vi "WeightingCheckNew.vi"() -> ()   [LabVIEW 2012]
uses:
  <vilib>/addons/database/Auxilliary.llb/DB Tools Cursor Type.ctl
  <vilib>/addons/database/Connection.llb/DB Tools Open Connec (Path).vi
  <vilib>/Utility/file.llb/Read From Spreadsheet File (string).vi
  <vilib>/addons/database/Connection.llb/Conn Execute.vi
  <vilib>/addons/database/Recordset.llb/Rec Fetch Integer Data (R).vi
  <vilib>/addons/database/Recordset.llb/Rec Destroy - Connection.vi
  <vilib>/Utility/file.llb/Write To Spreadsheet File (string).vi
  <vilib>/addons/database/NI_Database_API.lvlib
panel:
  out "WrongDate":bool
  in  "Cluster":T1
  out "after substring":string
  out "Wrong RC":bool
  out "STD Weight Check":bool
  out "Total Check":bool
  out "data":i32
  out "Pass Check":bool
  out "ProdLine":bool
  out "error out":errorcluster
  out "filenames":string[](array[string])
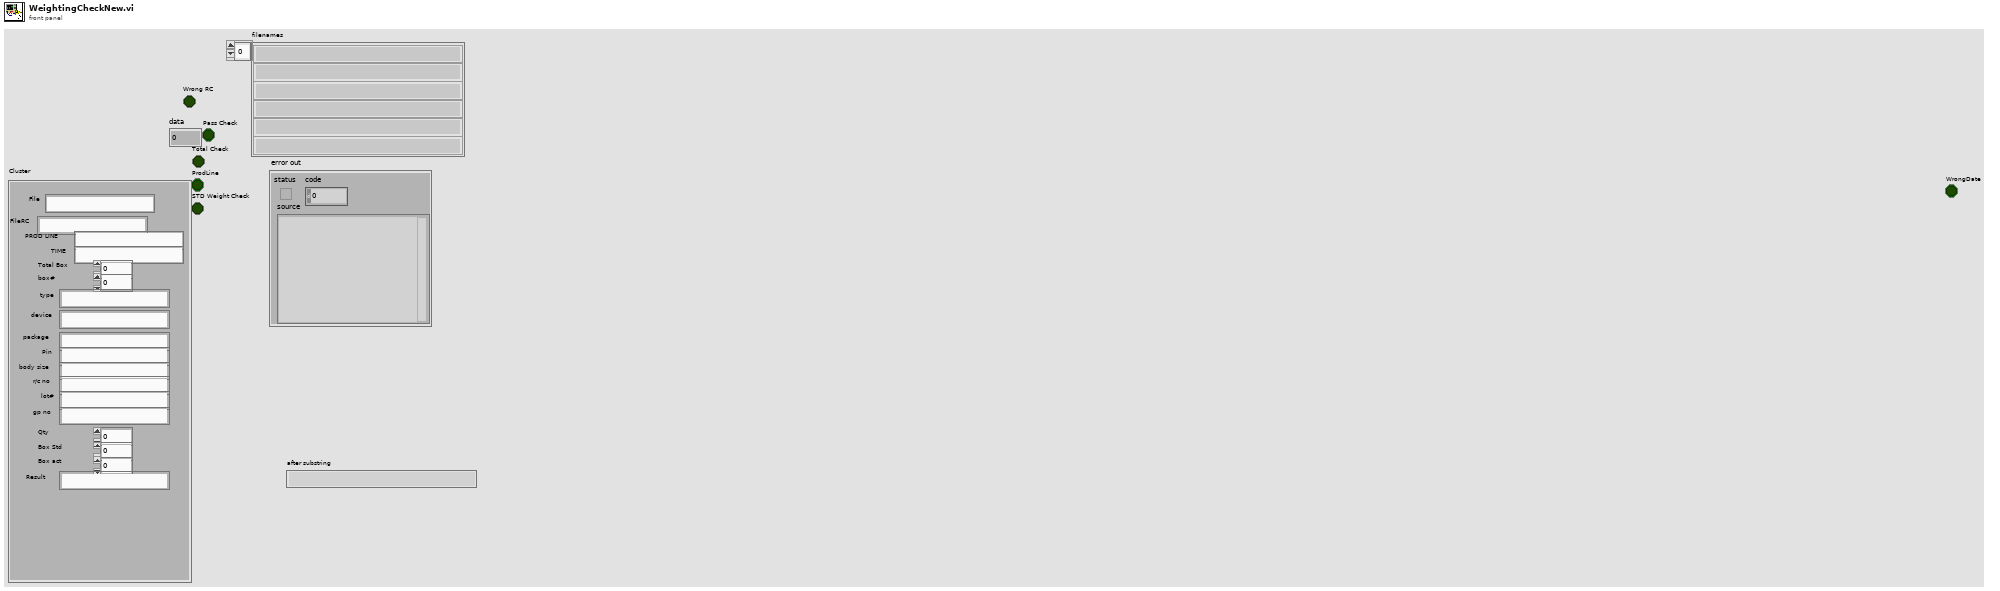
[diagram p1: front panel]
types:
  T1 = cluster{"File":string, "FileRC":string, "PROD LINE ":string, "TIME":string, "Total Box":dbl, "box#":dbl, "type":string, "device":string, "package":string, "Pin ":string, "body size":string, "r/c no":string, "lot#":string, "gp no":string, "Qty":dbl, "Box Std":dbl, "Box act":dbl, "Result":string}
  T2 = typedef "NI_Database_API.lvlib/DB Tools Cursor Type.ctl" = enum16{"forward-only", "keyset", "dynamic", "static"}
  T3 = typedef "NI_Database_API.lvlib/Conn ObjectReference.ctl" = refnum<k1>
  T4 = typedef "NI_Database_API.lvlib/Rec ObjectReference.ctl" = refnum<k1>
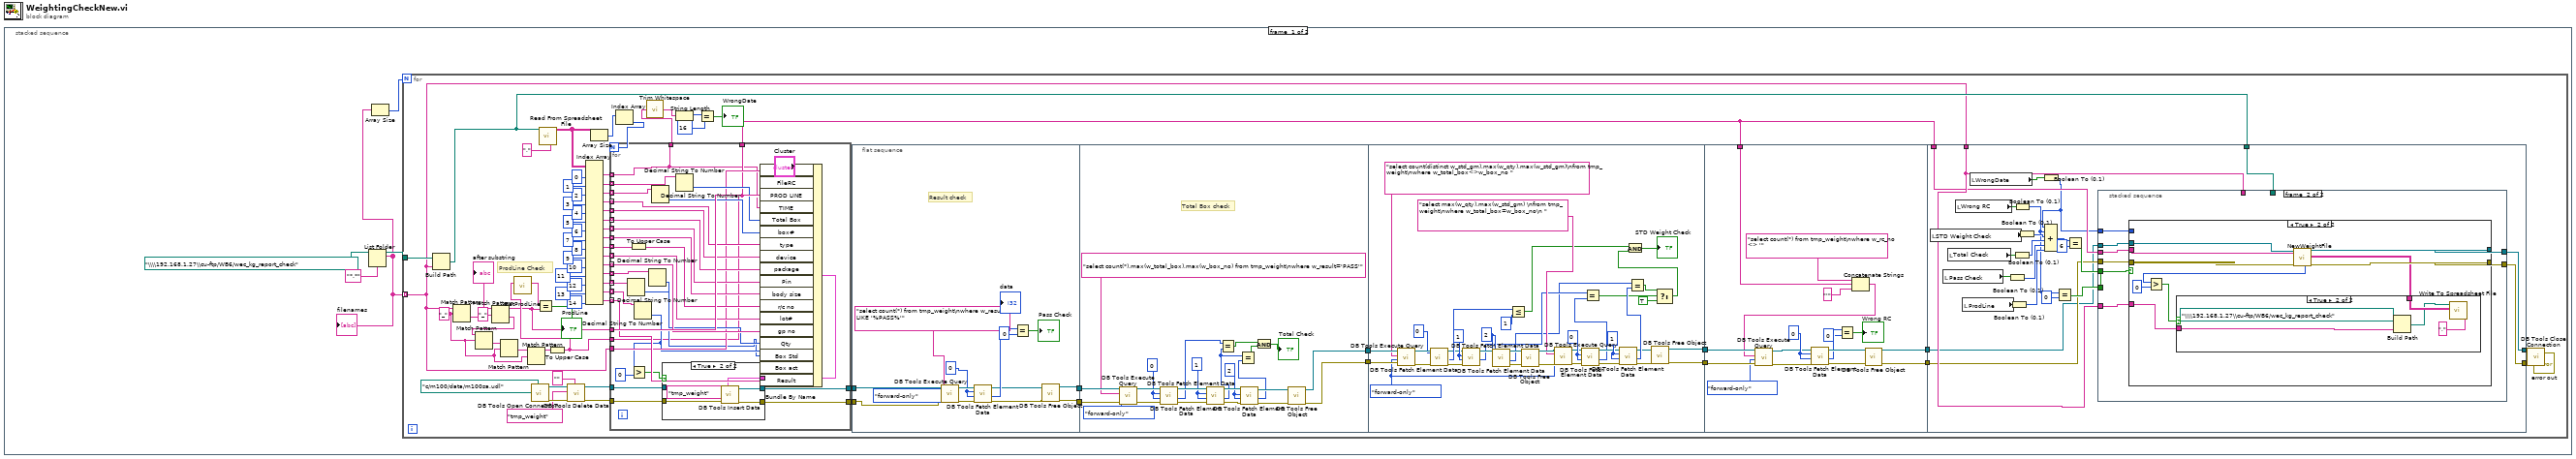
[diagram p0: block diagram]
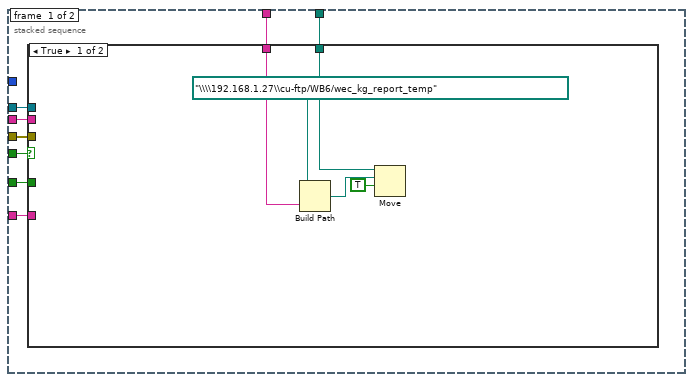
[diagram p2: hidden frame]
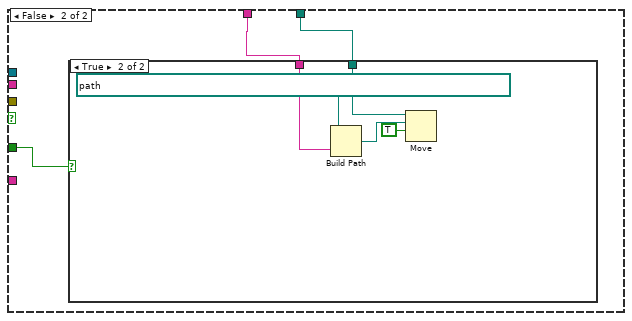
[diagram p3: hidden frame]
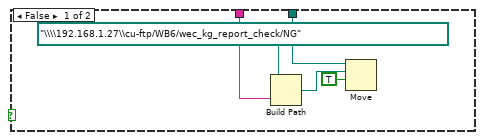
[diagram p4: hidden frame]
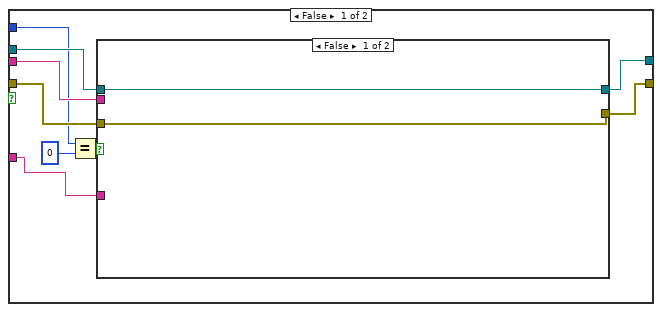
[diagram p5: hidden frame]
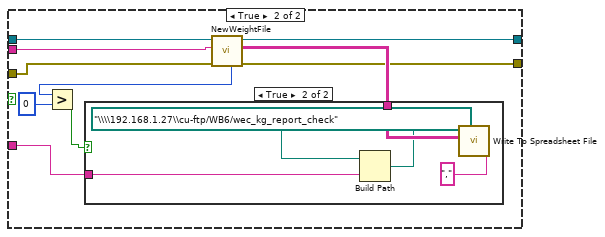
[diagram p6: hidden frame]
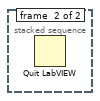
[diagram p10: hidden frame]
diagram:
  n1 = stacked-sequence {
    frame #0 {
      n2 = List Folder(path=path "\\\\192.168.1.27\\cu-ftp/WB6/wec_kg_report_check", pattern="*.*") -> (path out=w3:path, filenames=w1:string[])  [unwired: 2 in, 2 out]
      "filenames" <- w1
      n3 = Array Size(array=w1) -> (size(s)=w2:i32)
      n4 = for {
        N: w2 -> [_]
        tunnel: w3 -> [w61]
        tunnel: w1 -> [w15] mode=indexing
        w56 = "_" ("regular expression")
        # "ProdLine Check"
        n5 = Build Path(base path=w61, name or relative path=w15) -> (appended path=w16:path)
        n6 = Match Pattern(string=w15, regular expression=w56) -> (after substring=w59:string)  [unwired: 1 in, 3 out]
        "after substring" <- w59
        n7 = Match Pattern(string=w59, regular expression="_") -> (before substring=w24:string, after substring=w55:string)  [unwired: 1 in, 2 out]
        n8 = Match Pattern(string=w55, regular expression=w56) -> (after substring=w58:string)  [unwired: 1 in, 3 out]
        n9 = Match Pattern(string=w58, regular expression=w56) -> (after substring=w57:string)  [unwired: 1 in, 3 out]
        n10 = Match Pattern(string=w57, regular expression=w56) -> (before substring=w54:string)  [unwired: 1 in, 3 out]
        n11 = call-poly <vilib>:"DB Tools Open Connection.vi"("connection information"=path "c:/m100/data/m100sa.udl") -> ("error out"=w35:errorcluster, "connection reference"=w36:T3)  [unwired: 7 in]
        n12 = call-poly <vilib>:"Read From Spreadsheet File.vi"("delimiter (\\t)"="," ("delimiter (\\t)"), "file path (dialog if empty)"=w16) -> ("all rows"=w77:string[][])  [unwired: 5 in, 4 out]
        n13 = To Upper Case(1:w54) -> (0:w26:string)
        n14 = call "GetProdLine.vi"("Lotno"=w26) -> ("ProdLine"=w25:string)  [unwired: 10 in]
        n15 = Equal?(x=w25, y=w24) -> (x = y?=→"ProdLine":bool)
        n16 = call <vilib>:"DB Tools Delete Data.vi"("condition"="", "error in (no error)"=w35, "table"="tmp_weight", "connection reference"=w36) -> ("error out"=w33:errorcluster, "connection reference out"=w34:T3)  [unwired: 6 in]
        n17 = Index Array(array=w77, index (col) #1=0 ("disabled index (col)"), index (col) #2=1 ("index (col)"), index (col) #3=2 ("index (col)"), index (col) #4=3 ("index (col)"), index (col) #5=4 ("index (col)"), index (col) #6=5 ("index (col)"), index (col) #7=6 ("index (col)"), index (col) #8=7 ("index (col)"), index (col) #9=8 ("index (col)"), index (col) #10=9 ("index (col)"), index (col) #11=10 ("index (col)"), index (col) #12=11 ("index (col)"), index (col) #13=12 ("index (col)"), index (col) #14=13 ("index (col)"), index (col) #15=14 ("index (col)")) -> (element #1=w69:string[], element #2=w67:string[], element #3=w66:string[], element #4=w65:string[], element #5=w64:string[], element #6=w63:string[], element #7=w62:string[], element #8=w47:string[], element #9=w44:string[], element #10=w43:string[], element #11=w42:string[], element #12=w41:string[], element #13=w40:string[], element #14=w39:string[], element #15=w38:string[])  [unwired: 15 in]
        n18 = Array Size(array=w77) -> (size(s)=w78:i32[])
        n19 = Index Array(array=w78) -> (element=w68:i32)  [unwired: 1 in]
        n20 = for {
          N: w68 -> [_]
          tunnel: w69 -> [w272] mode=indexing
          tunnel: w67 -> [w302] mode=indexing
          tunnel: w66 -> [w298] mode=indexing
          tunnel: w65 -> [w296] mode=indexing
          tunnel: w64 -> [w295] mode=indexing
          tunnel: w63 -> [w294] mode=indexing
          tunnel: w62 -> [w293] mode=indexing
          tunnel: w47 -> [w292] mode=indexing
          tunnel: w44 -> [w303] mode=indexing
          tunnel: w43 -> [w290] mode=indexing
          tunnel: w42 -> [w289] mode=indexing
          tunnel: w41 -> [w288] mode=indexing
          tunnel: w40 -> [w286] mode=indexing
          tunnel: w39 -> [w285] mode=indexing
          tunnel: w38 -> [w284] mode=indexing
          tunnel: w26 -> [w273]
          tunnel: w15 -> [w283]
          tunnel: w24 -> [w300]
          tunnel: w34 -> [w282]
          tunnel: w33 -> [w281]
          tunnel: [w280] -> w30
          tunnel: [w279] -> w29
          tunnel: [w273] -> w12
          tunnel: [w272] -> w6
          n21 = Decimal String To Number(string=w286) -> (number=w274:i32)  [unwired: 2 in, 1 out]
          n22 = To Upper Case(1:w303) -> (0:w291:string)
          n23 = Decimal String To Number(string=w285) -> (number=w277:i32)  [unwired: 2 in, 1 out]
          n24 = Greater?(x=w277, y=0) -> (0:w275:bool)
          n25 = Decimal String To Number(string=w288) -> (number=w287:i32)  [unwired: 2 in, 1 out]
          n26 = Decimal String To Number(string=w298) -> (number=w297:i32)  [unwired: 2 in, 1 out]
          n27 = Decimal String To Number(string=w302) -> (number=w299:i32)  [unwired: 2 in, 1 out]
          n28 = Bundle By Name(cluster="Cluster", "File"=w283, "FileRC"=w273, "PROD LINE"=w300, "TIME"=w272, "Total Box"=w299, "box#"=w297, "type"=w296, "device"=w295, "package"=w294, "Pin"=w293, "body size"=w292, "r/c no"=w291, "lot#"=w290, "gp no"=w289, "Qty"=w287, "Box Std"=w274, "Box act"=w277, "Result"=w284) -> (w278:T1)
          n29 = case shown="True" w275 {
            tunnel: w282 -> [w305 w311]
            tunnel: w281 -> [w304 w310]
            tunnel: [w305 w309] -> w280
            tunnel: [w304 w308] -> w279
            tunnel: w278 -> [_ w307]
            frame False {
            }
            frame True {
              n30 = call <vilib>:"DB Tools Insert Data.vi"("data"=w307, "error in (no error)"=w310, "table"="tmp_weight", "connection reference"=w311) -> ("error out"=w308:errorcluster, "connection reference out"=w309:T3)  [unwired: 6 in]
            }
          }
        }
        n31 = call <vilib>:"Trim Whitespace.vi"("string"=w6) -> ("trimmed string"=w7:string)  [unwired: 1 in]
        n32 = String Length(string=w7) -> (length=w10:i32)
        n33 = Equal?(x=w10, y=16) -> (x = y?=→"WrongDate":bool)
        n34 = flat-sequence {
          tunnel: w30 -> [w93]
          tunnel: [w83] -> w28
          tunnel: w29 -> [w92]
          tunnel: [w82] -> w27
          tunnel: w28 -> [w116]
          tunnel: w27 -> [w115]
          tunnel: [w112] -> w22
          tunnel: [w111] -> w21
          tunnel: w22 -> [w155]
          tunnel: w21 -> [w154]
          tunnel: [w118] -> w20
          tunnel: [w117] -> w19
          tunnel: w20 -> [w172]
          tunnel: w19 -> [w171]
          tunnel: w12 -> [w168]
          tunnel: [w161] -> w18
          tunnel: [w159] -> w17
          tunnel: w18 -> [w176]
          tunnel: w17 -> [w178]
          tunnel: w16 -> [w183]
          tunnel: w15 -> [w179]
          tunnel: [w181] -> w14
          tunnel: [w180] -> w13
          tunnel: w12 -> [w177]
          frame #0 {
            w87 = 0
            # "Result check"
            n35 = call-poly <vilib>:"DB Tools Execute Query.vi"("error in (no error)"=w92, "cursor type"=DB_Tools_Cursor_Type."forward-only", "SQL query"="select count(*) from tmp_weight\nwhere w_result NOT LIKE '%PASS%'", "connection reference"=w93) -> ("error out"=w91:errorcluster, "recordset reference"=w88:T4)  [unwired: 4 in]
            n36 = call-poly <vilib>:"DB Tools Fetch Element Data.vi"("error in (no error)"=w91, "type"=w87, "column index"=w87, "recordset reference"=w88) -> ("error out"=w80:errorcluster, "data"=w86:i32, "recordset reference out"=w81:T4)  [unwired: 3 in]
            "data" <- w86
            n37 = Equal?(x=w86, y=0) -> (x = y?=→"Pass Check":bool)
            n38 = call-poly <vilib>:"DB Tools Free Object.vi"("error in (no error)"=w80, "recordset reference"=w81) -> ("error out"=w82:errorcluster, "connection reference"=w83:T3)  [unwired: 8 in]
          }
          frame #1 {
            w99 = 2
            w105 = 1
            w108 = 0
            # "Total Box check"
            n39 = call-poly <vilib>:"DB Tools Execute Query.vi"("error in (no error)"=w115, "cursor type"=DB_Tools_Cursor_Type."forward-only", "SQL query"="select count(*),max(w_total_box),max(w_box_no) from tmp_weight\nwhere w_result='PASS'", "connection reference"=w116) -> ("error out"=w113:errorcluster, "recordset reference"=w114:T4)  [unwired: 4 in]
            n40 = call-poly <vilib>:"DB Tools Fetch Element Data.vi"("error in (no error)"=w113, "type"=w108, "column index"=w108, "recordset reference"=w114) -> ("error out"=w106:errorcluster, "data"=w104:i32, "recordset reference out"=w107:T4)  [unwired: 3 in]
            n41 = call-poly <vilib>:"DB Tools Fetch Element Data.vi"("error in (no error)"=w106, "type"=w105, "column index"=w105, "recordset reference"=w107) -> ("error out"=w101:errorcluster, "data"=w98:i32, "recordset reference out"=w103:T4)  [unwired: 3 in]
            n42 = Equal?(x=w104, y=w98) -> (x = y?=w95:bool)
            n43 = call-poly <vilib>:"DB Tools Fetch Element Data.vi"("error in (no error)"=w101, "type"=w99, "column index"=w99, "recordset reference"=w103) -> ("error out"=w100:errorcluster, "data"=w97:i32, "recordset reference out"=w102:T4)  [unwired: 3 in]
            n44 = Equal?(x=w98, y=w97) -> (x = y?=w96:bool)
            n45 = And(x=w95, y=w96) -> (x .and. y?=→"Total Check":bool)
            n46 = call-poly <vilib>:"DB Tools Free Object.vi"("error in (no error)"=w100, "recordset reference"=w102) -> ("error out"=w111:errorcluster, "connection reference"=w112:T3)  [unwired: 8 in]
          }
          frame #2 {
            w139 = 1
            w140 = 0
            w143 = 2
            w147 = 1
            w150 = 0
            w132 = DB_Tools_Cursor_Type."forward-only" ("cursor type")
            n47 = call-poly <vilib>:"DB Tools Execute Query.vi"("error in (no error)"=w154, "cursor type"=w132, "SQL query"="select count(distinct w_std_gm),max(w_qty),max(w_std_gm)\nfrom tmp_weight\nwhere w_total_box<>w_box_no ", "connection reference"=w155) -> ("error out"=w152:errorcluster, "recordset reference"=w153:T4)  [unwired: 4 in]
            n48 = call-poly <vilib>:"DB Tools Fetch Element Data.vi"("error in (no error)"=w152, "type"=w150, "column index"=w150, "recordset reference"=w153) -> ("error out"=w145:errorcluster, "data"=w149:i32, "recordset reference out"=w146:T4)  [unwired: 3 in]
            n49 = call-poly <vilib>:"DB Tools Fetch Element Data.vi"("error in (no error)"=w145, "type"=w147, "column index"=w147, "recordset reference"=w146) -> ("data"=w130:i32, "recordset reference out"=w144:T4)  [unwired: 3 in, 1 out]
            n50 = call-poly <vilib>:"DB Tools Fetch Element Data.vi"("type"=w143, "column index"=w143, "recordset reference"=w144) -> ("error out"=w141:errorcluster, "data"=w128:i32, "recordset reference out"=w142:T4)  [unwired: 4 in]
            n51 = Less Or Equal?(x=w149, y=1) -> (x <= y?=w123:bool)
            n52 = call-poly <vilib>:"DB Tools Free Object.vi"("error in (no error)"=w141, "recordset reference"=w142) -> ("error out"=w133:errorcluster, "connection reference"=w134:T3)  [unwired: 8 in]
            n53 = call-poly <vilib>:"DB Tools Execute Query.vi"("error in (no error)"=w133, "cursor type"=w132, "SQL query"="select max(w_qty),max(w_std_gm) \nfrom tmp_weight\nwhere w_total_box=w_box_no\n ", "connection reference"=w134) -> ("error out"=w135:errorcluster, "recordset reference"=w136:T4)  [unwired: 4 in]
            n54 = call-poly <vilib>:"DB Tools Fetch Element Data.vi"("error in (no error)"=w135, "type"=w140, "column index"=w140, "recordset reference"=w136) -> ("error out"=w137:errorcluster, "data"=w129:i32, "recordset reference out"=w138:T4)  [unwired: 3 in]
            n55 = Equal?(x=w130, y=w129) -> (x = y?=w126:bool)
            n56 = call-poly <vilib>:"DB Tools Fetch Element Data.vi"("error in (no error)"=w137, "type"=w139, "column index"=w139, "recordset reference"=w138) -> ("error out"=w119:errorcluster, "data"=w127:i32, "recordset reference out"=w120:T4)  [unwired: 3 in]
            n57 = Equal?(x=w128, y=w127) -> (x = y?=w125:bool)
            n58 = call-poly <vilib>:"DB Tools Free Object.vi"("error in (no error)"=w119, "recordset reference"=w120) -> ("error out"=w117:errorcluster, "connection reference"=w118:T3)  [unwired: 8 in]
            n59 = Select(t=w125, s=w126, f=TRUE) -> (s? t:f=w122:bool)
            n60 = And(x=w123, y=w122) -> (x .and. y?=→"STD Weight Check":bool)
          }
          frame #3 {
            w165 = 0
            n61 = Concatenate Strings("select count(*) from tmp_weight\nwhere w_rc_no <> '", w168, "'") -> (w166:string)
            n62 = call-poly <vilib>:"DB Tools Execute Query.vi"("error in (no error)"=w171, "cursor type"=DB_Tools_Cursor_Type."forward-only", "SQL query"=w166, "connection reference"=w172) -> ("error out"=w163:errorcluster, "recordset reference"=w164:T4)  [unwired: 4 in]
            n63 = call-poly <vilib>:"DB Tools Fetch Element Data.vi"("error in (no error)"=w163, "type"=w165, "column index"=w165, "recordset reference"=w164) -> ("error out"=w160:errorcluster, "data"=w158:i32, "recordset reference out"=w162:T4)  [unwired: 3 in]
            n64 = Equal?(x=w158, y=0) -> (x = y?=→"Wrong RC":bool)
            n65 = call-poly <vilib>:"DB Tools Free Object.vi"("error in (no error)"=w160, "recordset reference"=w162) -> ("error out"=w159:errorcluster, "connection reference"=w161:T3)  [unwired: 8 in]
          }
          frame #4 {
            n66 = local read "STD Weight Check"() -> (w195:bool)
            n67 = local read "Pass Check"() -> (w193:bool)
            n68 = local read "Total Check"() -> (w194:bool)
            n69 = local read "Wrong RC"() -> (w196:bool)
            n70 = local read "ProdLine"() -> (w192:bool)
            n71 = local read "WrongDate"() -> (w173:bool)
            n72 = Boolean To (0,1)(Boolean=w193) -> (0, 1=w189:i16)
            n73 = Boolean To (0,1)(Boolean=w192) -> (0, 1=w188:i16)
            n74 = Boolean To (0,1)(Boolean=w194) -> (0, 1=w190:i16)
            n75 = Boolean To (0,1)(Boolean=w196) -> (0, 1=w175:i16)
            n76 = Boolean To (0,1)(Boolean=w195) -> (0, 1=w191:i16)
            n77 = Boolean To (0,1)(Boolean=w173) -> (0, 1=w174:i16)
            n78 = Compound Arithmetic op=ADD(w174, w175, w191, w190, w189, w188) -> (w187:i16)
            n79 = Equal?(x=w175, y=i16 0) -> (x = y?=w182:bool)
            n80 = Equal?(x=w187, y=i16 6) -> (x = y?=w185:bool)
            n81 = stacked-sequence {
              tunnel: w185 -> [w204 _]
              tunnel: w179 -> [w203 _]
              tunnel: w183 -> [w202 _]
              tunnel: w182 -> [w201 w228]
              tunnel: [_ w230] -> w181
              tunnel: [_ w229] -> w180
              tunnel: w179 -> [w197 w227]
              tunnel: w178 -> [w198 w226]
              tunnel: w177 -> [w199 w225]
              tunnel: w176 -> [w200 w224]
              tunnel: w174 -> [_ w223]
              frame #0 {
                n82 = case shown="True" w204 {
                  tunnel: w202 -> [w209 w212]
                  tunnel: w203 -> [w206 w211]
                  tunnel: w201 -> [_ w210]
                  tunnel: w200 -> [_ _]
                  tunnel: w199 -> [_ _]
                  tunnel: w198 -> [_ _]
                  tunnel: w197 -> [_ _]
                  frame True {
                    n83 = Build Path(base path=path "\\\\192.168.1.27\\cu-ftp/WB6/wec_kg_report_temp", name or relative path=w206) -> (appended path=w208:path)
                    n84 = Move(source path=w209, 9:TRUE ("overwrite (F)"), 10:w208) -> ()  [unwired: 2 in, 3 out]
                  }
                  frame False {
                    n85 = case shown="True" w210 {
                      tunnel: w212 -> [w217 w222]
                      tunnel: w211 -> [w214 w219]
                      frame False {
                        n86 = Build Path(base path=path "\\\\192.168.1.27\\cu-ftp/WB6/wec_kg_report_check/NG", name or relative path=w214) -> (appended path=w216:path)
                        n87 = Move(source path=w217, 9:TRUE ("overwrite (F)"), 10:w216) -> ()  [unwired: 2 in, 3 out]
                      }
                      frame True {
                        n88 = Build Path(base path=path "\\\\192.168.1.27\\cu-ftp/WB6/wec_kg_report_check/修正前", name or relative path=w219) -> (appended path=w221:path)
                        n89 = Move(source path=w222, 9:TRUE ("overwrite (F)"), 10:w221) -> ()  [unwired: 2 in, 3 out]
                      }
                    }
                  }
                }
              }
              frame #1 {
                n90 = case shown="True" w228 {
                  tunnel: w224 -> [w239 w266]
                  tunnel: w226 -> [w238 w265]
                  tunnel: [w237 w264] -> w230
                  tunnel: [w236 w263] -> w229
                  tunnel: w227 -> [w234 w262]
                  tunnel: w225 -> [w235 w261]
                  tunnel: w223 -> [w232 _]
                  frame False {
                    n91 = Equal?(x=w232, y=i16 0) -> (x = y?=w233:bool)
                    n92 = case shown="False" w233 {
                      tunnel: w239 -> [w241 w250]
                      tunnel: w238 -> [w240 w249]
                      tunnel: [w241 w248] -> w237
                      tunnel: [w240 w247] -> w236
                      tunnel: w235 -> [_ w246]
                      tunnel: w234 -> [_ w245]
                      frame False {
                      }
                      frame True {
                        n93 = call "NewWeightFile.vi"("error in (no error)"=w249, "RC No"=w246, "connection reference"=w250) -> ("error out"=w247:errorcluster, "Array"=w251:string[][], "connection reference out"=w248:T3, "Numeric"=w244:i32)  [unwired: 5 in]
                        n94 = Greater?(x=w244, y=0) -> (0:w242:bool)
                        n95 = case shown="True" w242 {
                          tunnel: w251 -> [_ w255]
                          tunnel: w245 -> [_ w252]
                          frame False {
                          }
                          frame True {
                            n96 = Build Path(base path=path "\\\\192.168.1.27\\cu-ftp/WB6/wec_kg_report_check", name or relative path=w252) -> (appended path=w254:path)
                            n97 = call-poly <vilib>:"Write To Spreadsheet File.vi"("delimiter (\\t)"="," ("delimiter (\\t)"), "2D data"=w255, "file path (dialog if empty)"=w254) -> ()  [unwired: 5 in, 1 out]
                          }
                        }
                      }
                    }
                  }
                  frame True {
                    n98 = call "NewWeightFile.vi"("error in (no error)"=w265, "RC No"=w261, "connection reference"=w266) -> ("error out"=w263:errorcluster, "Array"=w260:string[][], "connection reference out"=w264:T3, "Numeric"=w259:i32)  [unwired: 5 in]
                    n99 = Greater?(x=w259, y=0) -> (0:w257:bool)
                    n100 = case shown="True" w257 {
                      tunnel: w262 -> [_ w271]
                      tunnel: w260 -> [_ w269]
                      frame False {
                      }
                      frame True {
                        n101 = Build Path(base path=path "\\\\192.168.1.27\\cu-ftp/WB6/wec_kg_report_check", name or relative path=w271) -> (appended path=w268:path)
                        n102 = call-poly <vilib>:"Write To Spreadsheet File.vi"("delimiter (\\t)"="," ("delimiter (\\t)"), "2D data"=w269, "file path (dialog if empty)"=w268) -> ()  [unwired: 5 in, 1 out]
                      }
                    }
                  }
                }
              }
            }
          }
        }
        n103 = call <vilib>:"DB Tools Close Connection.vi"("error in (no error)"=w13, "connection reference"=w14) -> ("error out"=→"error out":errorcluster)  [unwired: 5 in]
      }
    }
    frame #1 {
      n104 = Quit LabVIEW() -> ()  [unwired: 1 in]
    }
  }
